vi "pulse_more.vi"(8 "错误输入（无错误）":errorcluster, 10 "pulse num":dbl, 11 "axie":enum16{"x", "y"}(ring)) -> (0 "错误输出":errorcluster)   [LabVIEW 2013]
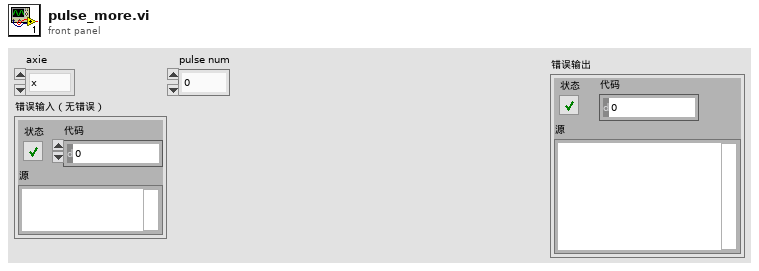
[diagram p1: front panel]
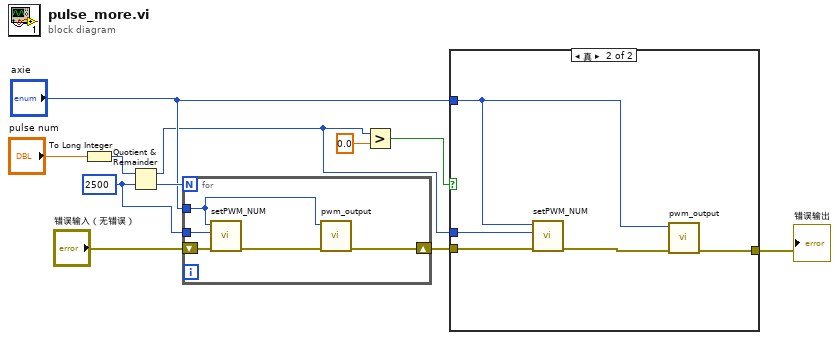
[diagram p0: block diagram]
diagram:
  w8 = 2500 ("y")
  n1 = To Long Integer(number="pulse num") -> (32bit integer=w10:i32)
  n2 = Quotient & Remainder(x=w10, y=w8) -> (x-y*floor(x/y)=w1:i32, floor(x/y)=w9:i32)
  n3 = for {
    N: w9 -> [_]
    tunnel: w8 -> [w15]
    shift-right: [w14] -> w6
    shift-left: "错误输入（无错误）" -> [w13]
    tunnel: "axie" -> [w12]
    n4 = call "setPWM_NUM.vi"("错误输入（无错误）"=w13, "pulse num"=w15, "axie"=w12) -> ("错误输出"=w16:errorcluster)  [unwired: 8 in]
    n5 = call "pwm_output.vi"("错误输入（无错误）"=w16, "axie"=w12) -> ("错误输出"=w14:errorcluster)  [unwired: 9 in]
  }
  n6 = Greater?(x=w1, y=0.0) -> (0:w2:bool)
  n7 = case shown="真" w2 {
    tunnel: w6 -> [w17 w21]
    tunnel: [w17 w20] -> w5
    tunnel: "axie" -> [_ w19]
    tunnel: w1 -> [_ w18]
    frame False {
    }
    frame True {
      n8 = call "setPWM_NUM.vi"("错误输入（无错误）"=w21, "pulse num"=w18, "axie"=w19) -> ("错误输出"=w22:errorcluster)  [unwired: 8 in]
      n9 = call "pwm_output.vi"("错误输入（无错误）"=w22, "axie"=w19) -> ("错误输出"=w20:errorcluster)  [unwired: 9 in]
    }
  }
  "错误输出" <- w5
